vi "Undistort Image (ARGB).vi"(4 "Crop to Valid Pixels? (Default: True)":bool=TRUE, 5 "Border Type (Default: Constant)":T2, 6 "Use Fixed Point Remapping (Default: False)":bool, 7 "ARGB Colour (Default: Black)":T1={"Alpha"=255, "RGB"=0}, 8 "error in (no error)":errorcluster, 9 "ARGB Image Destination in":T3, 10 "ARGB Image Source in":T3, 11 "Image Undistorter in":refnum<class "Image Undistorter.lvclass">) -> (0 "error out":errorcluster, 2 "ARGB Image Destination":T3, 3 "Image Undistorter":refnum<class "Image Undistorter.lvclass">)   [LabVIEW 2020, in "image.lvlib" / "Image Undistorter.lvclass"]
doc: "Undistort the Source Image. The Destination image will be sized to fit."
uses:
  Image Undistorter.lvclass
  ARGB Image.ctl
  Border Type.ctl
  ARGB Colour.ctl
  Image Undistorter.lvclass/Image Undistorter.ctl
  ccc224f2-fea8-4097-85c8-c2b3fe04188f.vi
  <vilib>/Utility/error.llb/Error Cluster From Error Code.vi
  image.lvlib
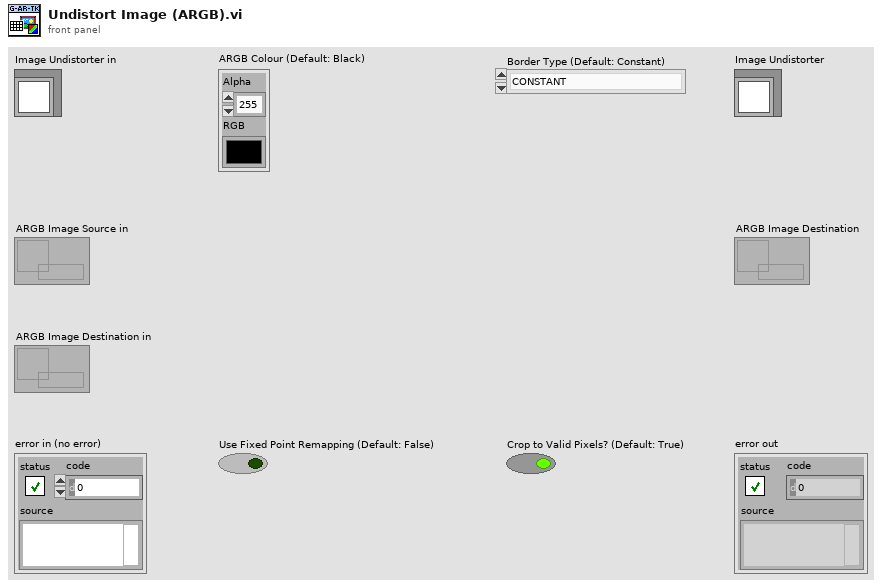
[diagram p1: front panel]
types:
  T1 = typedef "image.lvlib/ARGB Colour.ctl" = cluster{"Alpha":u8, "RGB":u32}
  T2 = typedef "image.lvlib/Border Type.ctl" = enum8{"CONSTANT", "REPLICATE", "REFLECT", "WRAP", "TRANSPARENT", "DEFAULT", "ISOLATED"}
  T3 = typedef "image.lvlib/ARGB Image.ctl" = refnum<data-value>
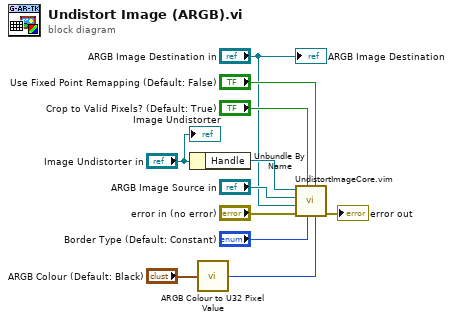
[diagram p0: block diagram]
diagram:
  n1 = Unbundle By Name("Image Undistorter in") -> ("Handle"=w10:refnum<data-value>)
  n2 = call "ARGB Colour to U32 Pixel Value.vi"("ARGB Colour"="ARGB Colour (Default: Black)") -> ("U32 Colour"=w1:u32)
  n3 = call "UndistortImageCore.vim"("Colour"=w1, "Use Fixed Point remapping"="Use Fixed Point Remapping (Default: False)", "Border Type"="Border Type (Default: Constant)", "Crop to Valid"="Crop to Valid Pixels? (Default: True)", "error in (no error)"="error in (no error)", "Destination Image"="ARGB Image Destination in", "Source Image"="ARGB Image Source in", "Handle"=w10) -> ("error out"=→"error out":errorcluster)  [unwired: 3 in]
  "Image Undistorter" <- "Image Undistorter in"
  "ARGB Image Destination" <- "ARGB Image Destination in"
